vi "Digital input.vi"(8 "error in":errorcluster, 11 "DAQmx InPut Setting":T1) -> (0 "error out":errorcluster, 1 "Exit":bool)   [LabVIEW 2015]
uses:
  <vilib>/DAQmx/read.llb/DAQmx Read (Digital 1D Bool 1Chan 1Samp).vi
  <vilib>/DAQmx/create/channels.llb/DAQmx Create Channel (DI-Digital Input).vi
  Galobal variable_TI.vi
  <vilib>/DAQmx/miscellaneous.llb/DAQmx Fill In Error Info.vi
panel:
  out "Boolean-01-Indicator":bool
  out "status":bool
  out "Array":bool[](array[boolean])
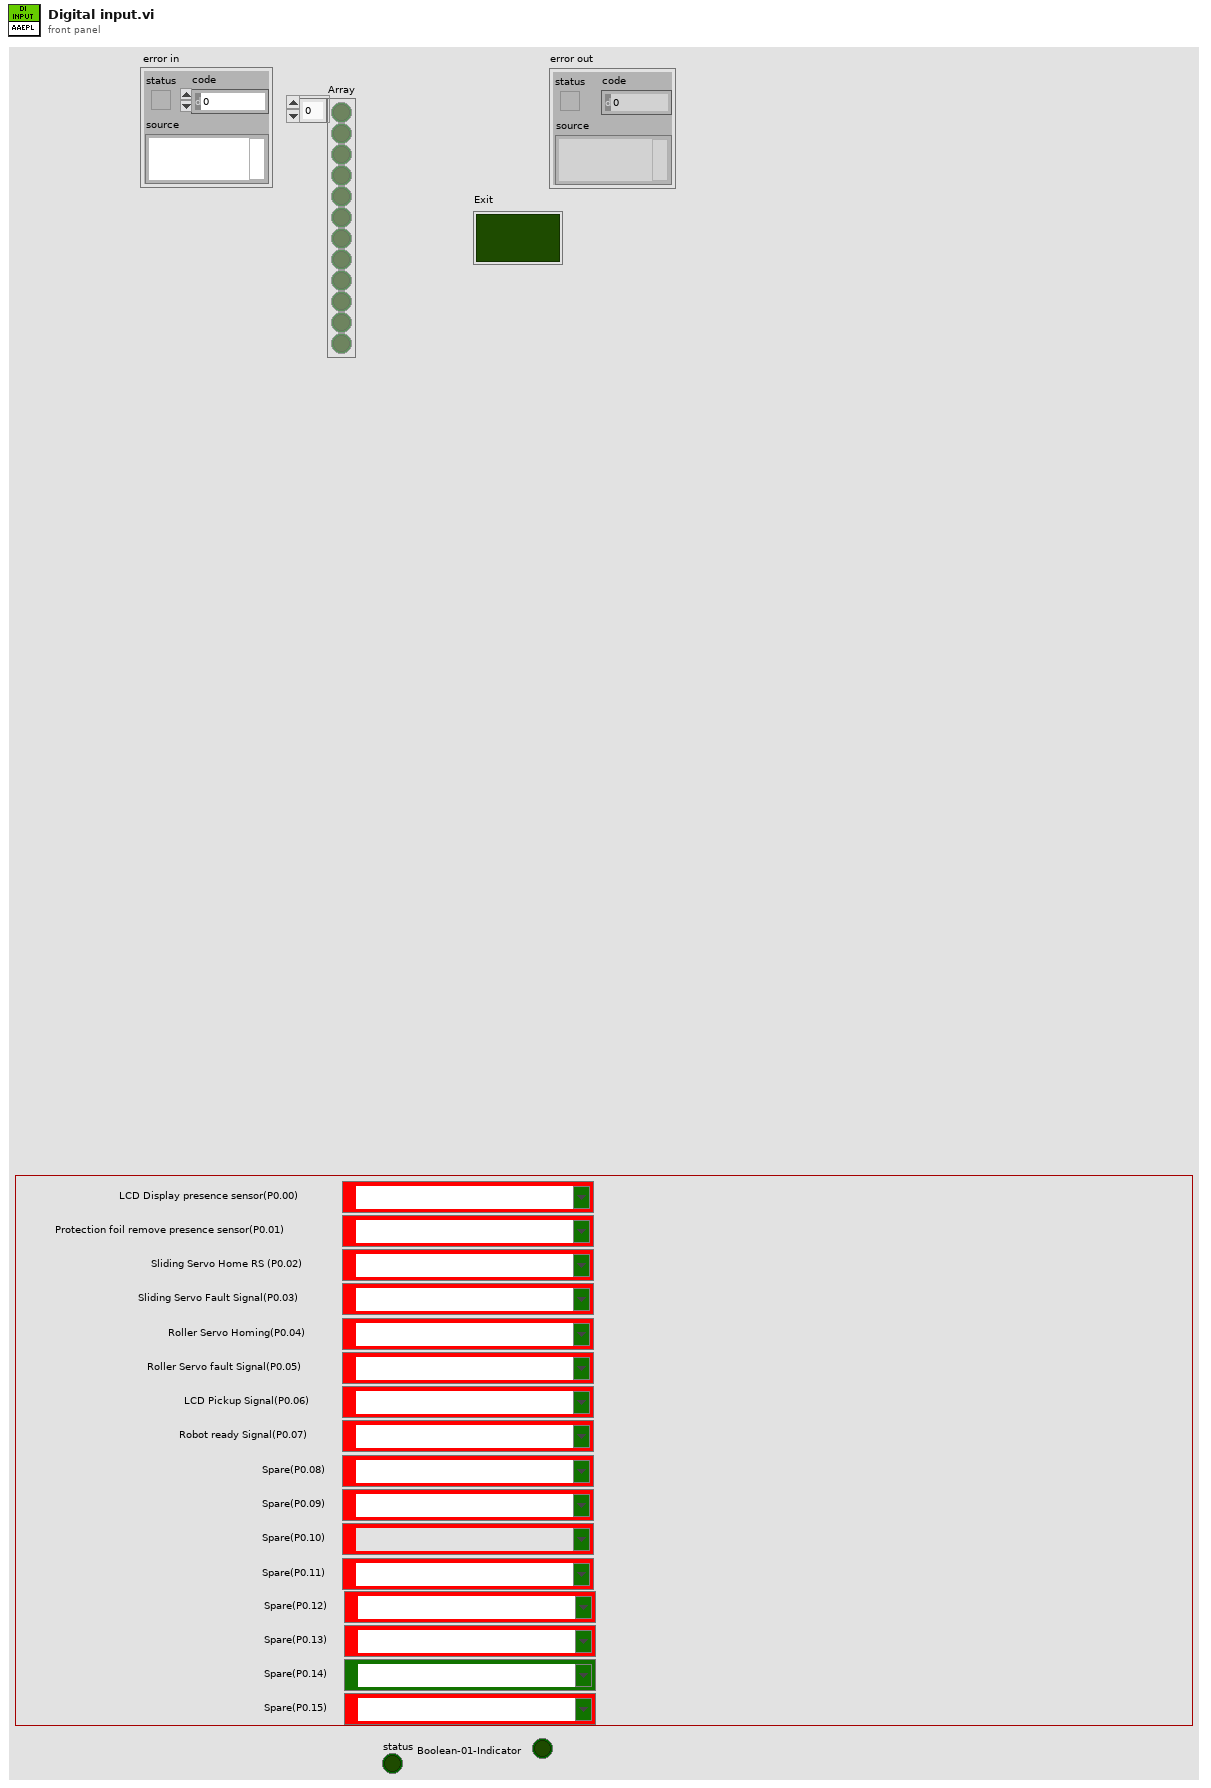
[diagram p1: front panel]
types:
  T1 = cluster{"DAQmx InPut_00":tag, "DAQmx InPut_01":tag, "DAQmx InPut_02":tag, "DAQmx InPut_03":tag, "DAQmx InPut_04":tag, "DAQmx InPut_05":tag, "DAQmx InPut_06":tag, "DAQmx InPut_07":tag, "DAQmx InPut_08":tag, "DAQmx InPut_09":tag, "DAQmx InPut_10":tag, "DAQmx InPut_11":tag, "DAQmx InPut_12":tag, "DAQmx InPut_13":tag, "DAQmx InPut_14":tag, "DAQmx InPut_15":tag}
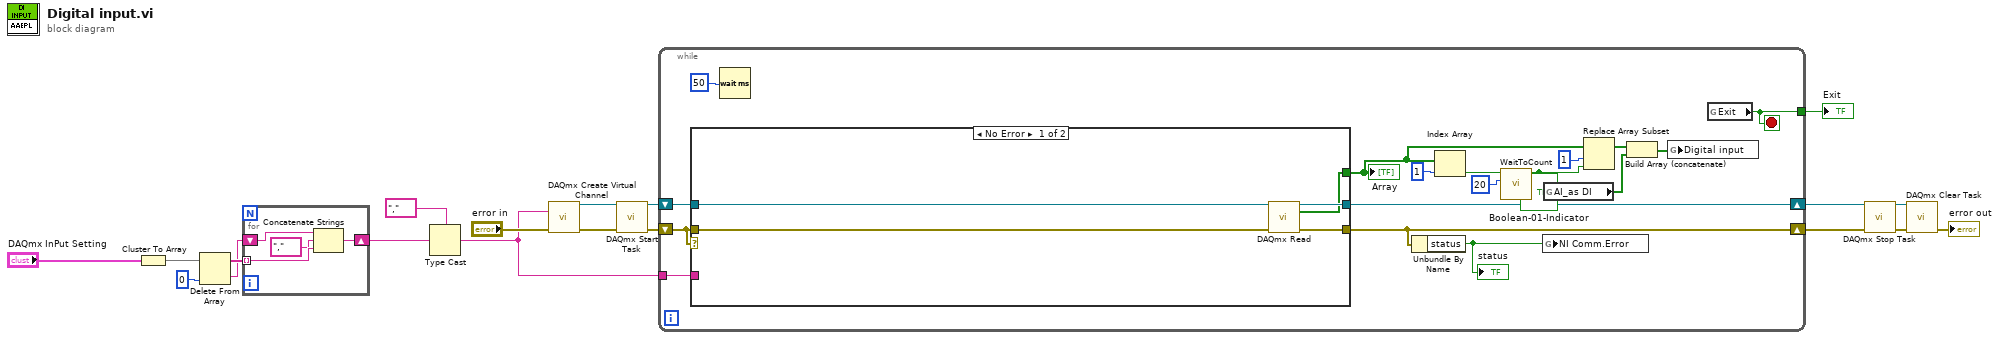
[diagram p0: block diagram]
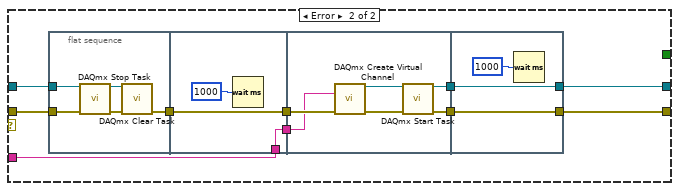
[diagram p2: hidden frame]
diagram:
  n1 = Cluster To Array(cluster="DAQmx InPut Setting") -> (array=w9:tag[])
  n2 = Delete From Array(array=w9, index=0) -> (deleted portion=w6:tag, array with subset deleted=w8:tag[])  [unwired: 1 in]
  n3 = for {
    tunnel: w8 -> [w22] mode=indexing
    shift-right: [w20] -> w4
    shift-left: w6 -> [w23]
    n4 = Concatenate Strings(w23, tag "," ("1."), w22) -> (w20:string)
  }
  n5 = Type Cast(type=tag "," ("1."), x=w4) -> (*(type *) &x=w3:tag)
  n6 = call-poly <vilib>:"DAQmx Create Virtual Channel.vi"("lines"=w3, "error in"="error in") -> ("task out"=w19:refnum<k21>, "error out"=w18:errorcluster)  [unwired: 3 in, 9 out]
  n7 = call <vilib>:"DAQmx Start Task.vi"("task/channels in"=w19, "error in"=w18) -> ("task out"=w16:refnum<k21>, "error out"=w17:errorcluster)  [unwired: 12 out]
  n8 = while {
    shift-right: [w33] -> w13
    shift-left: w17 -> [w40]
    shift-right: [w38] -> w12
    shift-left: w16 -> [w39]
    tunnel: w3 -> [w37]
    tunnel: [w36] -> w10
    stop <- w36 stop-if-true
    n9 = case shown="No Error" w40 {
      tunnel: w40 -> [w45 w54]
      tunnel: w39 -> [w44 w55]
      tunnel: [w43 w47] -> w33
      tunnel: [w42 w46] -> w38
      tunnel: w37 -> [_ w50]
      tunnel: [w41 _] -> w27
      frame No Error {
        n10 = call-poly <vilib>:"DAQmx Read.vi"("task/channels in"=w44, "error in"=w45) -> ("task out"=w42:refnum<k21>, "data"=w41:bool[], "error out"=w43:errorcluster)  [unwired: 1 in, 10 out]
      }
      frame Error {
        n11 = flat-sequence {
          tunnel: w55 -> [w58]
          tunnel: w54 -> [w57]
          tunnel: [w56] -> w53
          tunnel: w53 -> [w62]
          tunnel: [w62] -> w52
          tunnel: [w61] -> w51
          tunnel: w50 -> [w61]
          tunnel: w52 -> [w67]
          tunnel: w51 -> [w66]
          tunnel: [w65] -> w49
          tunnel: [w64] -> w48
          tunnel: w49 -> [w72]
          tunnel: w48 -> [w71]
          tunnel: [w72] -> w47
          tunnel: [w71] -> w46
          frame #0 {
            n12 = call <vilib>:"DAQmx Stop Task.vi"("task/channels in"=w58, "error in"=w57) -> ("task out"=w59:refnum<k21>, "error out"=w60:errorcluster)  [unwired: 12 in]
            n13 = call <vilib>:"DAQmx Clear Task.vi"("task in"=w59, "error in"=w60) -> ("error out"=w56:errorcluster)  [unwired: 13 in]
          }
          frame #1 {
            n14 = Wait (ms)(milliseconds to wait=u32 1000) -> ()  [unwired: 1 out]
          }
          frame #2 {
            n15 = call-poly <vilib>:"DAQmx Create Virtual Channel.vi"("lines"=w66, "error in"=w67) -> ("task out"=w68:refnum<k21>, "error out"=w69:errorcluster)  [unwired: 3 in, 9 out]
            n16 = call <vilib>:"DAQmx Start Task.vi"("task/channels in"=w68, "error in"=w69) -> ("task out"=w64:refnum<k21>, "error out"=w65:errorcluster)  [unwired: 12 out]
          }
          frame #3 {
            n17 = Wait (ms)(milliseconds to wait=u32 1000) -> ()  [unwired: 1 out]
          }
        }
      }
    }
    "Array" <- w27
    n18 = Wait (ms)(milliseconds to wait=u32 50) -> ()  [unwired: 1 out]
    n19 = Unbundle By Name(w33) -> ("status"=w32:bool)
    "status" <- w32
    n20 = Index Array(array=w27, index=1) -> (element=w28:bool)
    n21 = call "WaitToCount.vi"("Count"=20, "Boolean-01"=w28) -> ("Boolean-01-Indicator"=w25:bool)  [unwired: 8 in, 1 out]
    "Boolean-01-Indicator" <- w25
    n22 = global write "Galobal variable_TI.vi" "NI Comm.Error"(w32) -> ()
    n23 = global read "Galobal variable_TI.vi" "AI_as DI"() -> (w34:bool[])
    n24 = Replace Array Subset(array=w27, new element=w25, index=1) -> (w24:bool[])
    n25 = Build Array (concatenate)(w24, w34) -> (w35:bool[])
    n26 = global write "Galobal variable_TI.vi" "Digital input"(w35) -> ()
    n27 = global read "Galobal variable_TI.vi" "Exit"() -> (w36:bool)
  }
  "Exit" <- w10
  n28 = call <vilib>:"DAQmx Stop Task.vi"("task/channels in"=w12, "error in"=w13) -> ("task out"=w14:refnum<k21>, "error out"=w15:errorcluster)  [unwired: 12 in]
  n29 = call <vilib>:"DAQmx Clear Task.vi"("task in"=w14, "error in"=w15) -> ("error out"=→"error out":errorcluster)  [unwired: 13 in]
